vi "curve fit.vi"() -> ()   [LabVIEW 2016]
uses:
  <vilib>/gmath/NI_Gmath.lvlib
  <vilib>/gmath/zero.llb/nD Nonlinear System Solver (Formula).vi
panel:
  out "Zeroes 2":dbl[][](array[numeric]) format="%0.2e"
  in  "F(X)":string[](array[string])
  out "ticks":u32
  out "Zeroes":dbl[][][](array[numeric]) format="%0.2e"
  in  "dy2 = 3*a*x2^2+2*b*x2+c":string
  in  "dy1 = 3*a*x1^2+2*b*x1+c":string
  in  "y2 = a*x2^3+b*x2^2+c*x2+d":string="a*3375+b*225+c*15+d-7"
  in  "y1 = a*x1^3+b*x1^2+c*x1+d":string
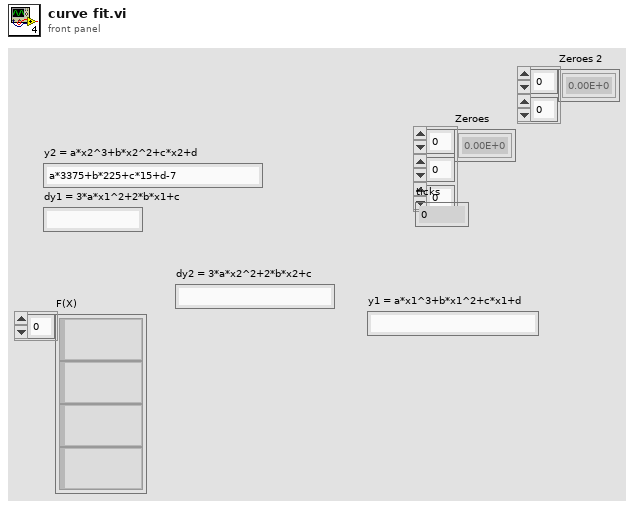
[diagram p1: front panel]
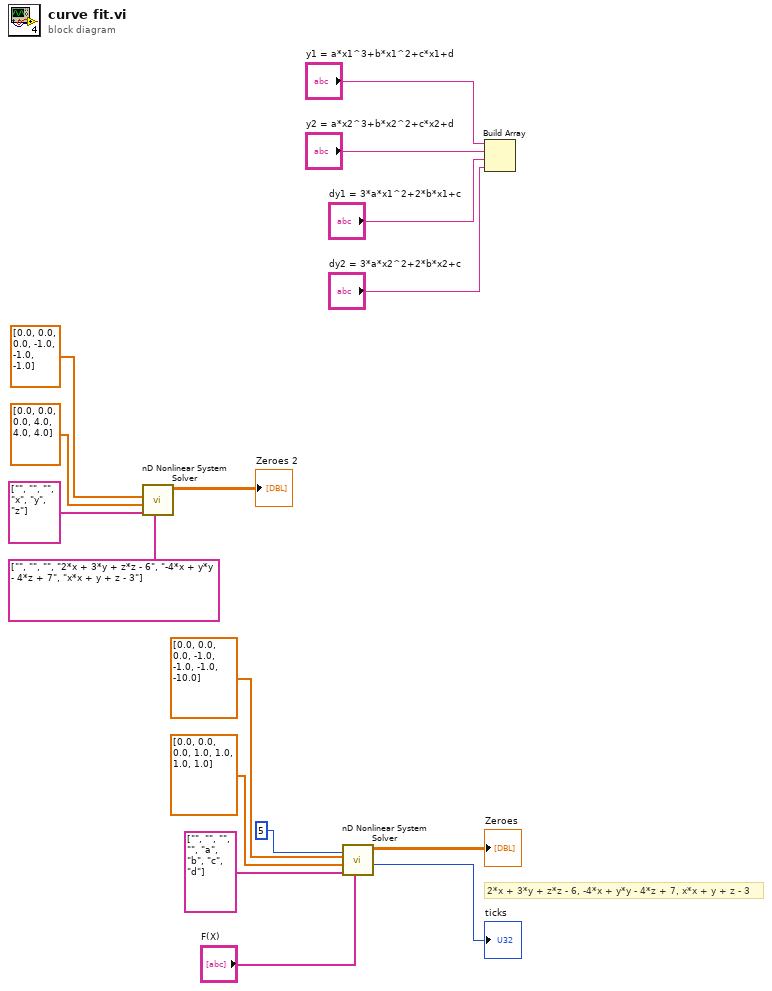
[diagram p0: block diagram]
diagram:
  # "2*x + 3*y + z*z - 6, -4*x + y*y - 4*z + 7, x*x + y + z - 3"
  n1 = call-poly <vilib>:"nD Nonlinear System Solver.vi"("F(X)"=string[] ["", "", "", "2*x + 3*y + z*z - 6", "-4*x + y*y - 4*z + 7", "x*x + y + z - 3"], "X"=string[] ["", "", "", "x", "y", "z"], "End"=dbl[] [0.0, 0.0, 0.0, 4.0, 4.0, 4.0], "Start"=dbl[] [0.0, 0.0, 0.0, -1.0, -1.0, -1.0]) -> ("Zeroes"=→"Zeroes 2":dbl[][])  [unwired: 4 in, 3 out]
  n2 = call-poly <vilib>:"nD Nonlinear System Solver.vi"("F(X)"="F(X)", "number of trials"=u32 5, "X"=string[] ["", "", "", "", "a", "b", "c", "d"], "End"=dbl[] [0.0, 0.0, 0.0, 1.0, 1.0, 1.0, 1.0], "Start"=dbl[] [0.0, 0.0, 0.0, -1.0, -1.0, -1.0, -10.0]) -> ("ticks"=→"ticks":u32, "Zeroes"=→"Zeroes":dbl[][])  [unwired: 3 in, 2 out]
  n3 = Build Array("y1 = a*x1^3+b*x1^2+c*x1+d", "y2 = a*x2^3+b*x2^2+c*x2+d", "dy1 = 3*a*x1^2+2*b*x1+c", "dy2 = 3*a*x2^2+2*b*x2+c") -> ()  [unwired: 1 out]
